vi "Check Internet Connectivity.vi"(8 "error in (no error)":errorcluster) -> (0 "error out":errorcluster, 3 "Connected To Internet?":bool)   [LabVIEW 2014]
doc: "This VI checks to see if the ground station has internet connectivity.\n\nTries to ping www.google.com\n\nReturns false if it can't see google."
panel:
  out "Status":i32(ring) items=["Success"=0, "DestinationNetworkUnreachable"=11002, "DestinationHostUnreachable"=11003, "DestinationProhibited, DestinationProtocolUnreachable"=11004, "DestinationPortUnreachable"=11005, "NoResources"=11006, "BadOption"=11007, "HardwareError"=11008, "PacketTooBig"=11009, "TimedOut"=11010, "BadRoute"=11012, "TtlExpired"=11013, "TtlReassemblyTimeExceeded"=11014, "ParameterProblem"=11015, "SourceQuench"=11016, "BadDestination"=11018, "DestinationUnreachable"=11040, "TimeExceeded"=11041, "BadHeader"=11042, "UnrecognizedNextHeader"=11043, "IcmpError"=11044, "DestinationScopeMismatch"=11045, "Unknown"=-1]
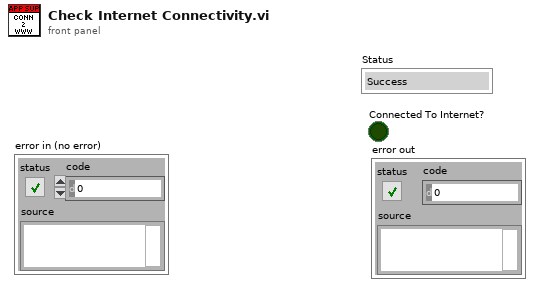
[diagram p1: front panel]
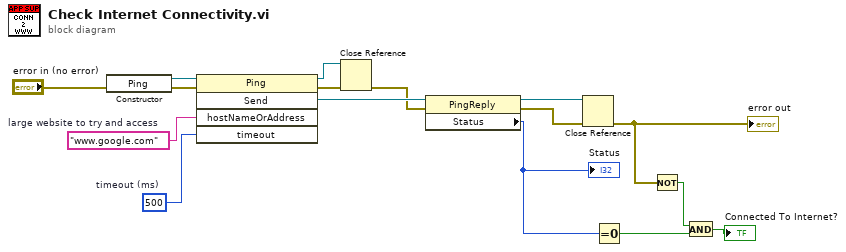
[diagram p0: block diagram]
diagram:
  w16 = 500  # timeout (ms)
  w14 = "www.google.com"  # large website to try and access
  n1 = constructor class="Ping"(error in="error in (no error)") -> (reference out=w13:refnum<k24>, error out=w7:errorcluster)  [unwired: 2 in, 1 out]
  n2 = invoke class="Ping" method="Send"(reference=w13, error in=w7, "hostNameOrAddress"=w14, "timeout"=w16) -> (reference out=w11:refnum<k24>, error out=w6:errorcluster, "Send"=w15:refnum<k24>)  [unwired: 1 in, 2 out]
  n3 = Close Reference(reference=w11, error in (no error)=w6) -> (error out=w5:errorcluster)
  n4 = property class="PingReply"(reference=w15, error in=w5) -> (reference out=w12:refnum<k24>, error out=w9:errorcluster, "Status"=w10:i32)
  "Status" <- w10
  n5 = Close Reference(reference=w12, error in (no error)=w9) -> (error out=w2:errorcluster)
  "error out" <- w2
  n6 = Equal To 0?(x=w10) -> (x = 0?=w4:bool)
  n7 = Not(x=w2) -> (.not. x?=w1:bool)
  n8 = And(x=w1, y=w4) -> (x .and. y?=→"Connected To Internet?":bool)
